vi "UI Main.vi"() -> ()   [LabVIEW 2018]
doc: "Main user interface VI running on HMI"
uses:
  Controls/Control Mode.ctl
  Controls/Parameters.ctl
  Controls/Sensor CalPara.ctl
  Controls/UI Controls.ctl
  Support/Message Queue/Message.ctl
  <vilib>/Utility/miscctls.llb/LVBoundsTypeDef.ctl
  Controls/Pumps Command.ctl
  Support/Message Queue/Message Cluster.ctl
  Controls/Calibration Cluster.ctl
  Controls/ConfigCalibration.ctl
  Controls/All Control Configuration Values.ctl
  Controls/Machine State.ctl
  Controls/TWT State.ctl
  Controls/OT State.ctl
  Controls/IT State.ctl
  Controls/BR State.ctl
  Controls/Pumps State.ctl
  Controls/DL State.ctl
  Controls/Clamp State.ctl
  Controls/Clean State.ctl
  Controls/Status Message.ctl
  Globals/Global - All UI Loop Stop.vi
  Globals/Global - UI Stream and Variable Connections.vi
  Globals/Global - Configuration Options.vi
  support/User Event - Stop/User Event - Stop.lvlib
  support/Message Queue/Message Queue.lvlib
panel:
  out "Temperature 8":u16(ring)
  out "Temperature 7":u16(ring)
  out "Temperature 6":u16(ring)
  in  "AB Valve":dbl(slide) scale=0.0..100.0
  in  "Horizontal Pointer Slide":dbl(slide) caption="Bleed Valve" scale=0.0..100.0
  in  "TC Valve":dbl(slide) scale=0.0..100.0
  out "Temp 11":dbl format="%.1f %"
  out "Pressure 7":dbl format="%.1f PSI"
  out "Temp 12":dbl format="%.1f F"
  out "Temp 10":dbl format="%.1f F"
  out "Pressure 5":dbl format="%.1f PSI"
  out "Temp 9":dbl format="%.1f F"
  out "RPM 2":dbl format="%.1f RPM"
  out "Temp 8":dbl format="%.1f F"
  out "Pressure 4":dbl format="%.1f PSI"
  out "Temp 7":dbl format="%.1f F"
  out "Temp 6":dbl format="%.1f F"
  out "Temp 5":dbl format="%.1f F"
  out "Temp 4":dbl format="%.1f F"
  out "Pressure 3":dbl format="%.1f PSI"
  out "Temp 3":dbl format="%.1f F"
  out "Temp 2":dbl format="%.1f F"
  in  "Checkbox 5":bool
  in  "Bearing Lube Switch 2":bool caption="Bearing Cooling"
  in  "Bearing Lube Switch":bool caption="Bearing Lube"
  out "RPM":dbl format="%.1f RPM"
  out "Pressure":dbl format="%.1f PSI"
  out "Temp":dbl format="%.1f F"
  in  "Checkbox 4":bool
  in  "Triplex Pump Switch":bool caption="Triplex Pump"
  in  "Oil Circ Switch":bool caption="Oil Circ"
  in  "Heater Switch":bool caption="Water Heater"
  out "Temperature 5":u16(ring)
  out "CRIO Version":string="V4.0" caption="CRIO:"
  out "HMI Version":string="V4.0" caption="HMI:"
  out "Temperature 2":u16(ring)
  in  "Tab Control":T1(tab)
  out "Pump 5":u16(ring)
  out "Pump 4":u16(ring)
  out "Pump 3":u16(ring)
  out "Pump 2":u16(ring)
  out "Oil Temperature Sid B (Deg F)":dbl(knob) scale=50.0..300.0 scale format="%#.1f"
  out "HPU Ambient\nTemperature (Deg F)":dbl(slide) scale=0.0..100.0 scale format="%#_1f"
  out "Oil Temperature Sid A (Deg F)":dbl(knob) scale=50.0..300.0 scale format="%#.1f"
  out "Pump 1":u16(ring)
  out "Temperature 3":u16(ring)
  out "Sensor CalPara":T2={"Body CalPara"={"Slope"=62500.0, "Intercept"=-250.0}, "US CalPara"={"Slope"=62500.0, "Intercept"=-250.0}} {"US CalPara"."Intercept" format="%.6f"; "US CalPara"."Slope" format="%.6f"; "Body CalPara"."Intercept" format="%.6f"; "Body CalPara"."Slope" format="%.6f"}
  in  "Stop":bool
  out "Running":bool
  out "Connection":bool
  out "data":T4
  out "Triplex Pump":bool
  out "Power Pack":bool
  out "Any Door":bool
  out "Platform Locks\nEngaged":bool
  out "Platform Locks\nDisengaged":bool
  out "Temperature 4":u16(ring)
  out "Mandrel Temp":dbl format="%.1f"
  out "Brg Mandrel Temp":dbl format="%.1f"
  out "Ambient Temp":dbl format="%.1f"
  out "Vessel Temp":dbl format="%.1f"
  out "Temperature":u16(ring)
  out "SW":dbl
  out "SE":dbl
  out "NW":dbl
  out "NE":dbl
  out "Cylinder Force (lbf)":cluster{i32, "number: 0 to 1":dbl}[](graph)
  in  "US CAL":bool caption="Sensor 1"
  in  "Body CAL":bool caption="Sensor 1"
  out "Free Memory (bytes)":dbl(graph)
  out "CPU Usage (%)":dbl(graph)
  in  "Status ListBox":i32(listbox)
  in  "Triplex Pump":dbl(slide) caption="Set Speed" scale=0.0..100.0
  # "Pressure Sensors"
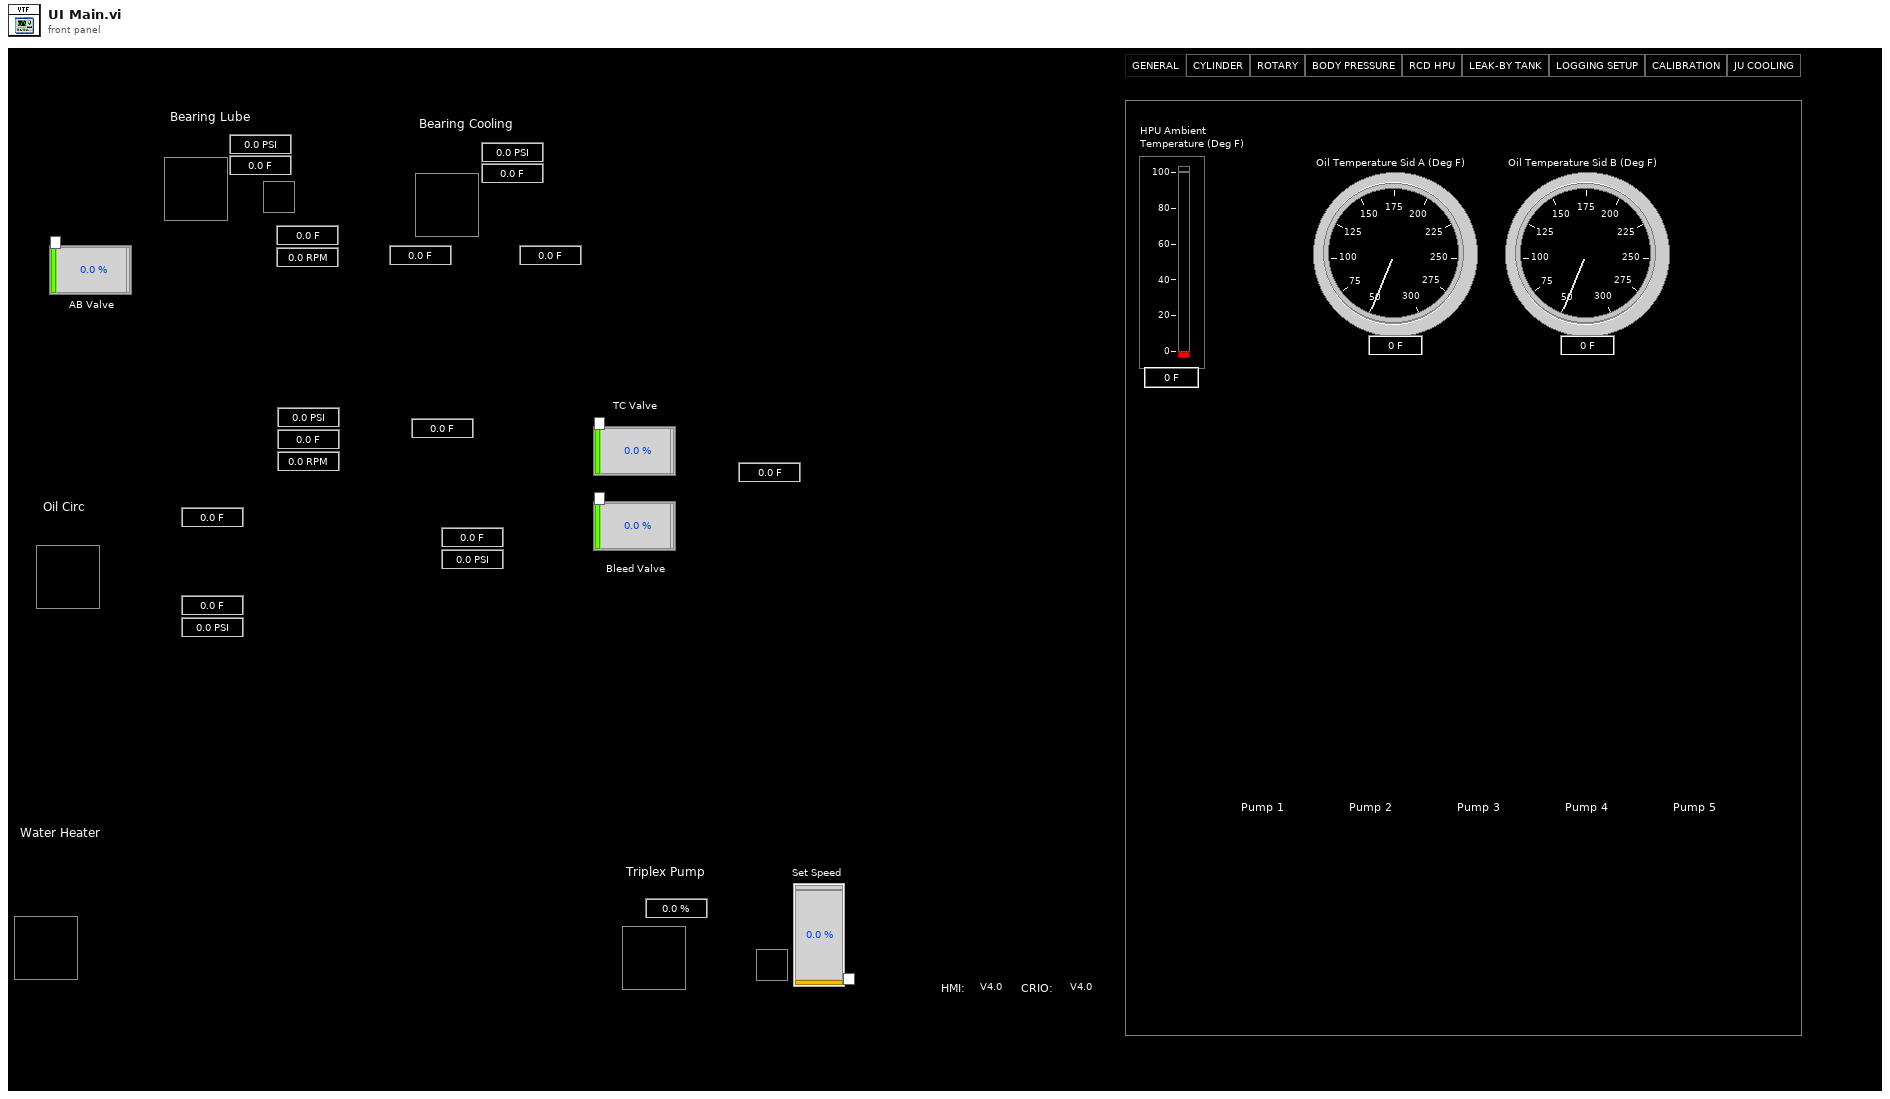
[diagram p1: front panel]
types:
  T1 = enum32{"GENERAL", "CYLINDER", "ROTARY", "BODY PRESSURE", "RCD HPU", "LEAK-BY TANK", "LOGGING SETUP", "CALIBRATION", "JU COOLING"}
  T2 = typedef "Parameters.ctl" = cluster{"Body CalPara":T3, "US CalPara":T3}
  T3 = typedef "Sensor CalPara.ctl" = cluster{"Slope":dbl, "Intercept":dbl}
  T4 = typedef "Control Mode.ctl" = enum16{"Skid Manual", "Computer Manual", "Step Automated", "Fully Automated"}
  T5 = typedef "UI Controls.ctl" = cluster{"Stop":refnum<vi>, "Pump 1":refnum<vi>, "Pump 2":refnum<vi>, "Pump 3":refnum<vi>, "Pump 4":refnum<vi>, "Pump 5":refnum<vi>}
  T6 = typedef "Message Queue.lvlib/All Message Queues.ctl" = cluster{"UI":refnum<queue>}
  T7 = typedef "Message Queue.lvlib/Message.ctl" = enum16{"Initialize", "Initialize UI Refs", "Disable Controls", "Enable UI Controls", "Connect RT", "Get Control Mode from RT", "Send Control Mode to UI", "Update Control Mode", "Get Config from RT", "Send Config to UI", "Update Parameters", "Change Parameters", "Calibrate Config", "Update Calibration", "Change Valve State", "Get Valve Status from RT", "Send Valve Status to UI", "Update Valve Status", "Inital UI Values", "Disconnect RT", "Close Connection", "Disconnect UI", "Run Mode", "Stop ALL", "Change Control Mode", "Skid Manual", "Computer Manual", "Step Automated", "Fully Automated", "Reset", "Pumps Command", "Pump State Changed", "Critical Error", "Log-Only Error", "Non-Critical Error", "RT Error", "Update System Status", "Update DI Status", "Clear System Status", "Update Warning", "Clear Warning", "Upate Timeout", "Update Reset Status", "Waiting", "Verify Password", "Manual Cleaning Process", "Update Manual Cleaning Process", "Cal - Body", "Cal - US", "Cal - Update Parameters", "Exit", "---Copy This Frame---"}
  T8 = typedef "LVBoundsTypeDef.ctl" = cluster{"Width":u32, "Height":u32}
  T9 = enum16{"Pump 1", "Pump 2", "Pump 3", "Pump 4", "Pump 5"}
  T10 = typedef "Pumps Command.ctl" = cluster{"Pump":enum16{"Pump 1", "Pump 2", "Pump 3", "Pump 4", "Pump 5"}, "Run/Stop":bool}
  T11 = enum8{"Enabled", "Disabled", "Disabled and Grayed Out"}
  T12 = typedef "Message Queue.lvlib/Message Cluster.ctl" = cluster{"Message":T7, "Message Data":variant}
  T13 = typedef "Calibration Cluster.ctl" = cluster{"CONFIG CALIBRATION":T14, "Calibration Value":dbl}
  T14 = typedef "ConfigCalibration.ctl" = enum16{"CAL STOP", "TWTT OP (IN)", "TWTT PDP (IN)", "DLT OP (IN)", "DLT PDP 01 (IN)", "DLT PDP 02 (IN)", "BR OP (IN)", "BR TWT ALIGN (IN)", "BR DL ALIGN (IN)"}
  T15 = typedef "All Control Configuration Values.ctl" = cluster{"MACHINE STATE":T16}
  T16 = typedef "Machine State.ctl" = cluster{"TWTT STATE":T17, "OT STATE":T18, "IT STATE":T19, "BR STATE":T20, "DLT STATE":T21, "DL STATE":T22, "CLAMP STATE":T23, "CLEAN STATE":T24}
  T17 = typedef "TWT State.ctl" = enum16{"TWTT STOP", "TWTT DRIVE FWD PDP", "TWTT DRIVE BWD PDP", "TWTT BWD 0.256 IN", "TWTT FWD 0.256 IN", "TWT FWD BEFORE SCREW", "SV-5 TWTT FWD TRUE", "SV-5 TWTT FWD FALSE", "SV-6 TWTT BWD TRUE", "SV-6 TWTT BWD FALSE", "TWTT RESET"}
  T18 = typedef "OT State.ctl" = enum16{"OT STOP", "OT ROTATE CW ENG", "OT ROTATE CCW 2.5 REV", "OT ROTATE CW 2.5 REV", "OT CW TIGHTEN PLUG", "SV-2 OT CW TRUE", "SV-2 OT CW FALSE", "SV-2 OT CCW TRUE", "SV-2 OT CCW FALSE"}
  T19 = typedef "IT State.ctl" = enum16{"IT STOP", "IT ROTATE CCW ENG", "IT ROTATE CCW QF1R", "IT CCW ENG & QF1R", "IT ROTATE CCW 2.5 REV", "IT ROTATE CW 2.5 REV", "IT CW TIGHTEN VALVE", "IT CCW PULSE", "SV-1 IT CW TRUE", "SV-1 IT CW FALSE", "SV-1 IT CCW TRUE", "SV-1 IT CCW FALSE"}
  T20 = typedef "BR State.ctl" = enum16{"BR STOP", "BR DRIVE LEFT PDP", "BR LEFT ALIGN TWT", "BR DRIVE RIGHT PDP", "BR RIGHT TO INIT", "BR RIGHT FOR DL", "SV-4 BR RIGHT TRUE", "SV-4 BR RIGHT FALSE", "SV-4 BR LEFT TRUE", "SV-4 BR LEFT FALSE", "BR RESET"}
  T21 = typedef "Pumps State.ctl" = enum16{"Do Nothing", "Run Pump 1", "Run Pump 2", "Run Pump 3", "Run Pump 4", "Run Pump 5", "Stop Pump 1", "Stop Pump 2", "Stop Pump 3", "Stop Pump 4", "Stop Pump 5"}
  T22 = typedef "DL State.ctl" = enum16{"DL STOP", "DL ROTATE CW", "DL ROTATE CCW", "SV-3 DL CW TRUE", "SV-3 DL CW FALSE", "SV-3 DL CCW TRUE", "SV-3 DL CCW FALSE"}
  T23 = typedef "Clamp State.ctl" = enum16{"CLAMP STOP", "CLAMP CLOSE", "CLAMP OPEN"}
  T24 = typedef "Clean State.ctl" = enum16{"CLEAN STOP", "CLEAN CAMERA", "CLEAN THREADS", "CLEAN THREADS MANUAL", "SV-12 H2O PILOT TRUE", "SV-12 H2O PILOT FALSE", "SV-13 CLEAN AIR TRUE", "SV-13 CLEAN AIR FALSE", "SV-15 CLEAN H2O TRUE", "SV-15 CLEAN H2O FALSE"}
  T25 = typedef "Status Message.ctl" = cluster{"Message":string, "Step #":i32, "Start/End":bool}
  T26 = cluster{"CPU Usage":refnum<k21>, "Contiguous Memory":refnum<k21>, "VTF Sensors":refnum<k21>}
  T27 = typedef "VTF Sensors.ctl" = cluster{"TJM Temp":dbl, "BrgM Temp":dbl, "Ambient Temp":dbl, "Vessel Temp":dbl}
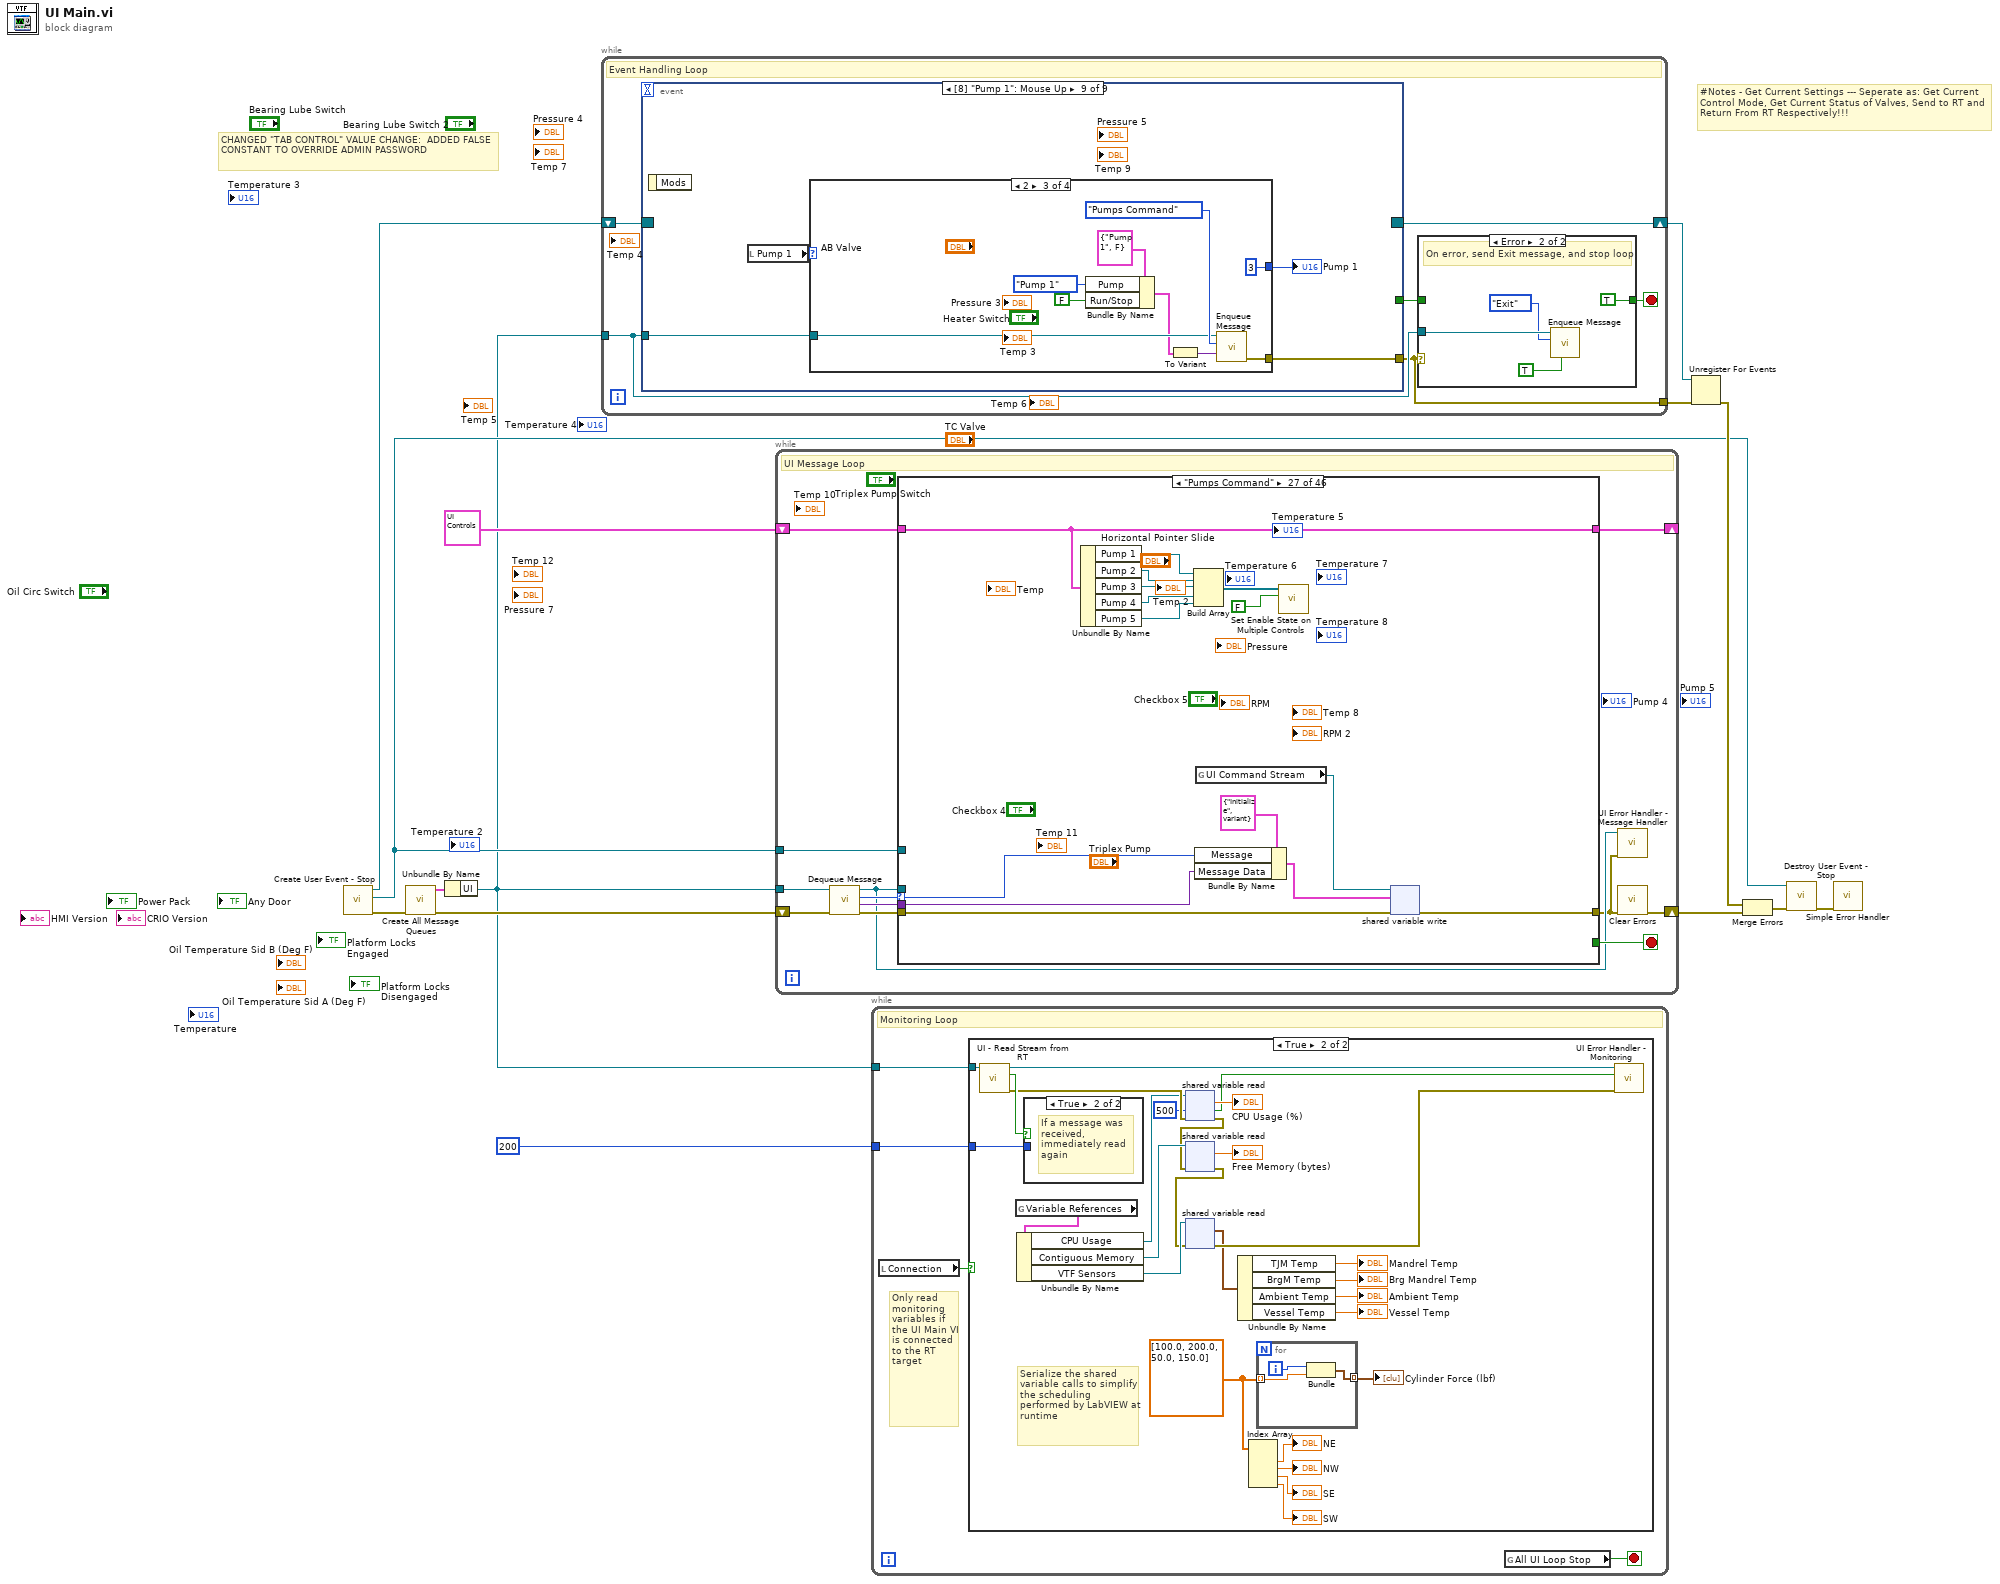
[diagram p0: block diagram]
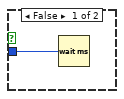
[diagram p3: hidden frame]
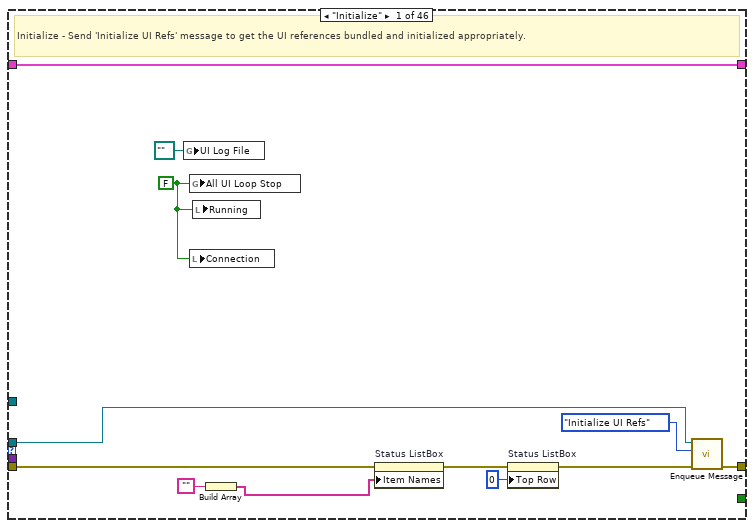
[diagram p4: hidden frame]
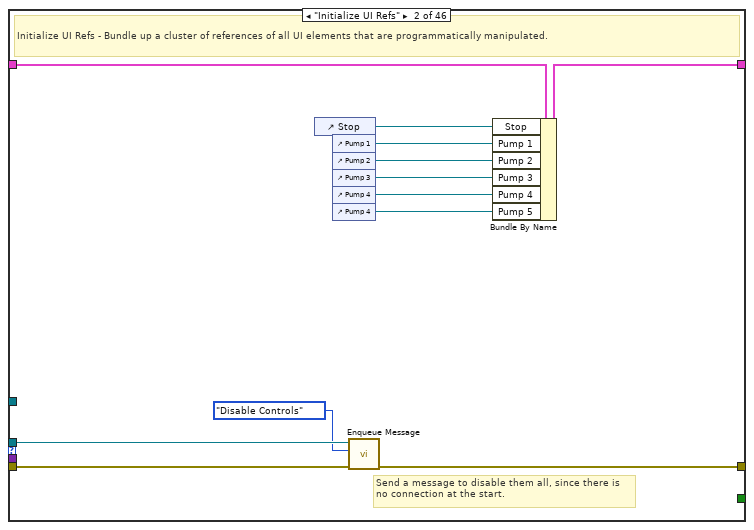
[diagram p5: hidden frame]
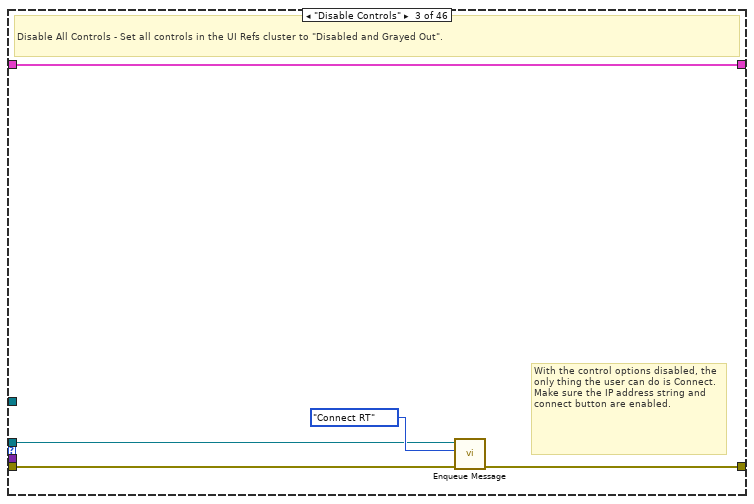
[diagram p6: hidden frame]
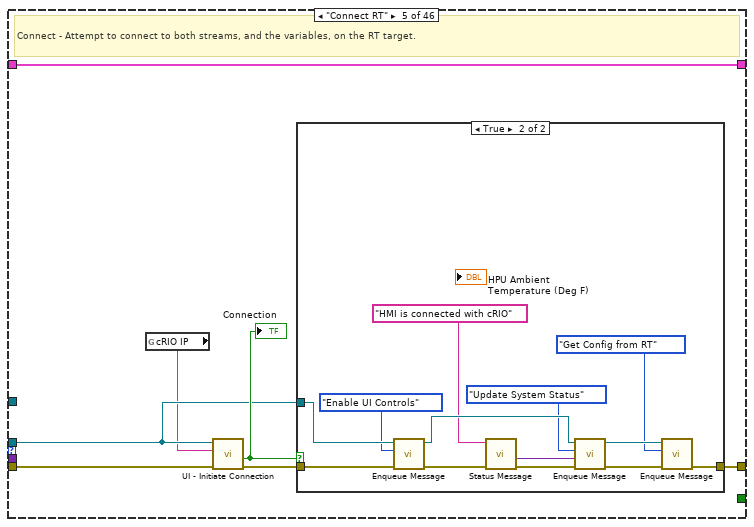
[diagram p8: hidden frame]
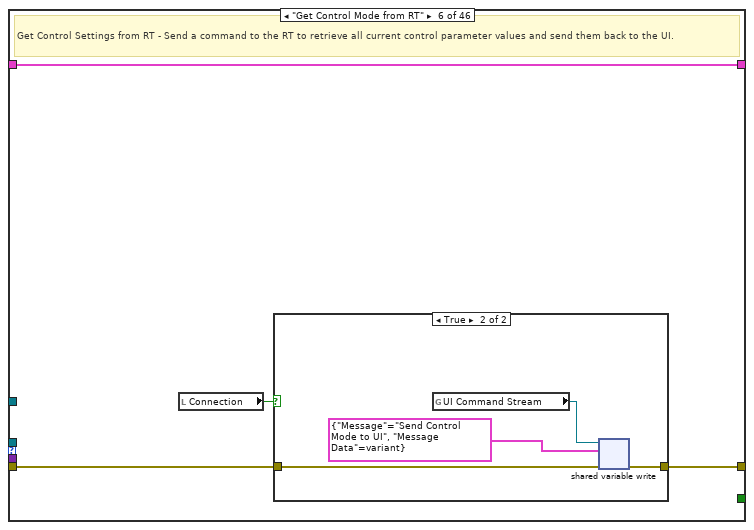
[diagram p10: hidden frame]
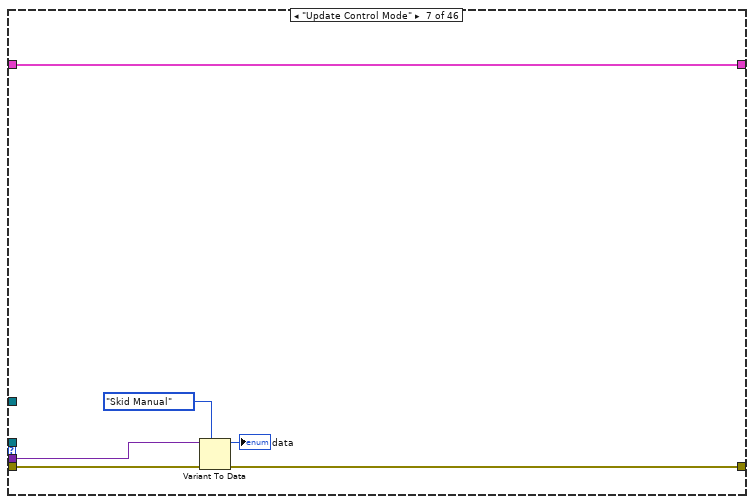
[diagram p12: hidden frame]
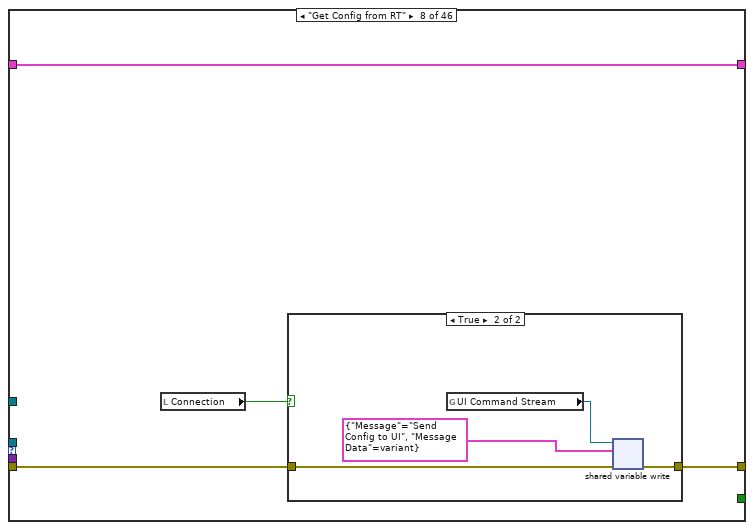
[diagram p13: hidden frame]
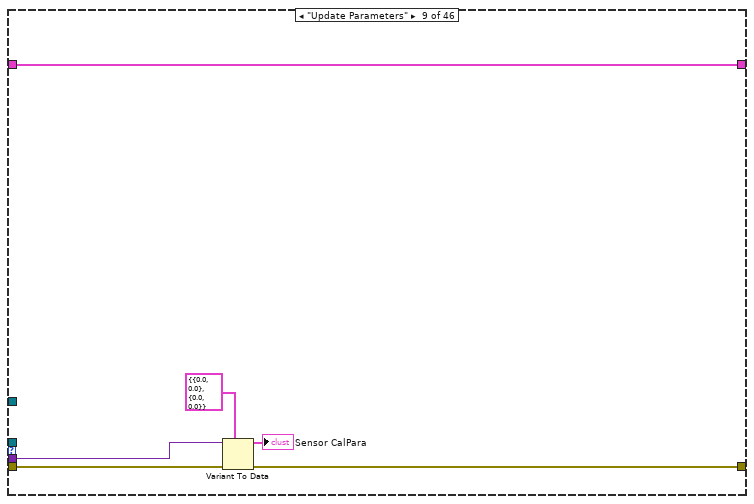
[diagram p15: hidden frame]
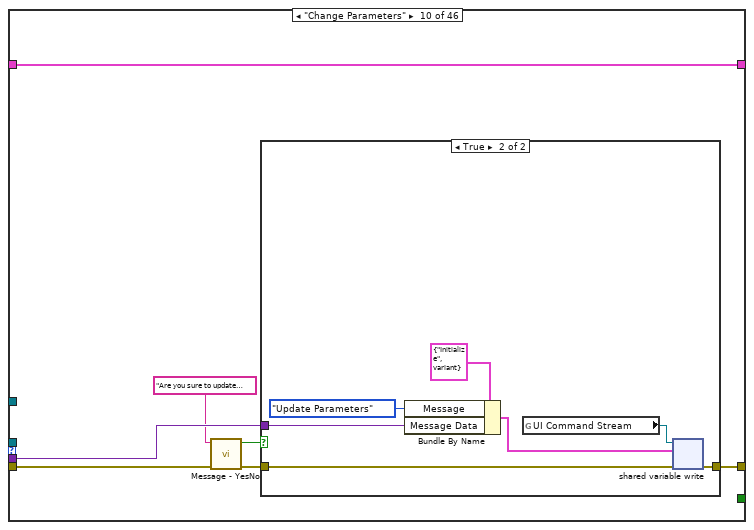
[diagram p16: hidden frame]
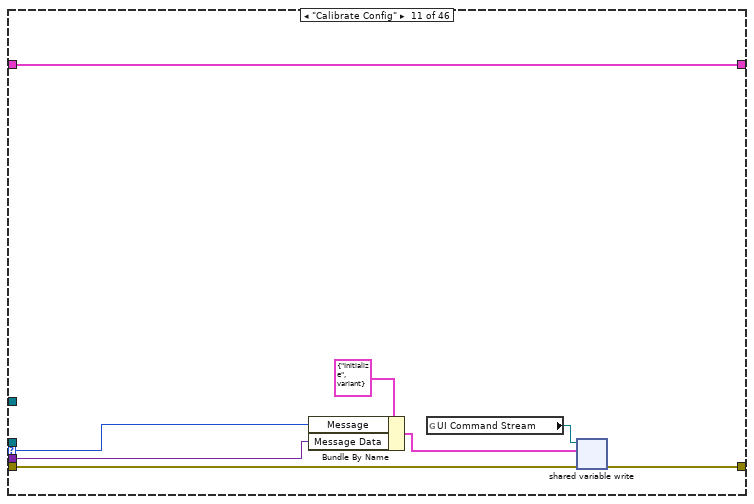
[diagram p18: hidden frame]
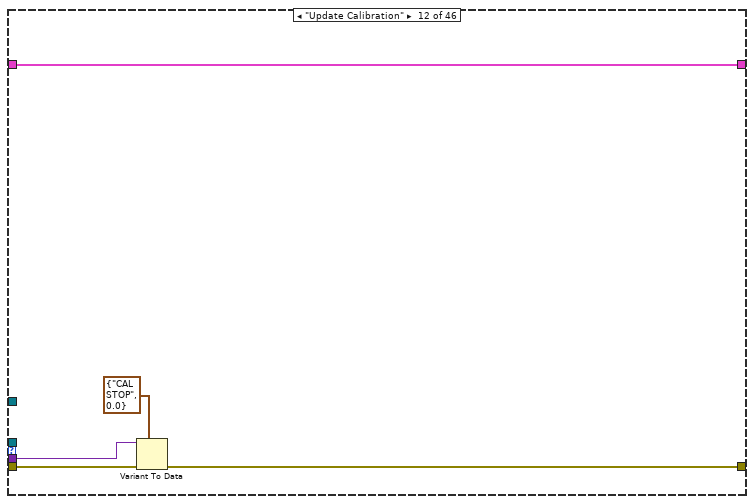
[diagram p19: hidden frame]
diagram:
  # "CHANGED \"TAB CONTROL\" VALUE CHANGE:  ADDED FALSE CONSTANT TO OVERRIDE ADMIN PASSWORD"
  # "#Notes - Get Current Settings --- Seperate as: Get Current Control Mode, Get Current Status of Valves, Send to RT and Return From RT Respectively!!!"
  n1 = call "Create User Event - Stop.vi"() -> ("error out"=w14:errorcluster, "User Event - Stop"=w3:refnum<user-event>, "Stop Event Registration Refnum"=w10:refnum<event-registration>)  [unwired: 9 in]
  n2 = call "Create All Message Queues.vi"("error in (no error)"=w14) -> ("error out"=w12:errorcluster, "Message Queues out"=w13:T6)  [unwired: 9 in]
  n3 = Unbundle By Name(w13) -> ("UI"=w1:refnum<queue>)
  n4 = while {
    tunnel: w1 -> [w20]
    tunnel: [w17] -> w8
    shift-right: [w15] -> w7
    shift-left: w10 -> [w16]
    stop <- w19 stop-if-true
    # "Event Handling Loop"
    n5 = event shown="[8] \"Pump 1\": Mouse Up" {
      selector: w16 -> [_ _ _ _ _ _ _ _ _]
      dyn-events: [_ _ _ _ _ _ _ _ _] -> w15
      timeout: _ -> [_ _ _ _ _ _ _ _ _]
      tunnel: w20 -> [w27 _ w47 _ _ _ w60 w63 w67]
      tunnel: [w26 w32 w46 _ _ _ w59 w62 w66] -> w17
      tunnel: [_ _ _ TRUE _ _ _ _ _] -> w18
      event "Stop": Value Change {
        n6 = event-data() -> ()  [unwired: 1 in, 1 out]
        n7 = call "Enqueue Message.vi"("Message"=Message."Stop ALL", "Message Queue"=w27) -> ("error out"=w26:errorcluster)  [unwired: 8 in, 1 out]
      }
      event "Tab Control": Value Change {
        n8 = event-data() -> ("CtlRef"=w31:refnum<vi>, "NewVal"=w29:T1)  [unwired: 1 in]
        n9 = property class="TabCtl (strict)"(reference=w31) -> (error out=w33:errorcluster, "Pages"=w30:refnum<vi>[])  [unwired: 1 in, 1 out]
        n10 = for {
          tunnel: w33 -> [w38]
          tunnel: [w37] -> w32
          tunnel: w30 -> [w35] mode=indexing
          tunnel: w29 -> [w34]
          i -> [w36]
          n11 = Equal?(x=w34, y=w36) -> (x = y?=w42:bool)
          n12 = Select(t=u32 0, s=w42, f=u32 6579300) -> (s? t:f=w39:u32)
          n13 = property class="Page"(reference=w35, error in=w38, "BG Color"=w39) -> (error out=w37:errorcluster)  [unwired: 1 out]
        }
      }
      event Panel Close? {
        w43 = TRUE  # Priority Message
        n14 = event-data() -> ()  [unwired: 1 in, 1 out]
        n15 = call "Enqueue Message.vi"("Priority Message? (F)"=w43, "Message"=Message."Exit", "Message Queue"=w47) -> ("error out"=w46:errorcluster)  [unwired: 7 in, 1 out]
        n16 = event-data("Discard?"=TRUE) -> ()  [unwired: 1 in, 1 out]
      }
      event User Event {
        # "The Message Handling Loop processed an \"Exit\" message, which fired this event to stop the Event Handling Loop."
        n17 = event-data() -> ()  [unwired: 1 in, 1 out]
      }
      event "Stop": Mouse Enter {
        n18 = event-data() -> ("CtlRef"=w51:refnum<vi>)  [unwired: 1 in]
        n19 = property class="Bool"(reference=w51) -> (reference out=w49:refnum<vi>, "DisabledEnum"=w50:T11)  [unwired: 1 in, 1 out]
        n20 = case shown="\"Enabled\", Default" w50 {
          tunnel: w49 -> [w52 _ _]
          frame "Enabled", Default {
            n21 = property class="Bool"(reference=w52, "Button Size"=T8 {"Width"=136, "Height"=57}) -> ()  [unwired: 1 in, 2 out]
          }
          frame "Disabled" {
          }
          frame "Disabled and Grayed Out" {
          }
        }
      }
      event "Stop": Mouse Leave {
        n22 = event-data() -> ("CtlRef"=w56:refnum<vi>)  [unwired: 1 in]
        n23 = property class="Bool"(reference=w56) -> (reference out=w54:refnum<vi>, "DisabledEnum"=w55:T11)  [unwired: 1 in, 1 out]
        n24 = case shown="\"Enabled\", Default" w55 {
          tunnel: w54 -> [w57 _ _]
          frame "Enabled", Default {
            n25 = property class="Bool"(reference=w57, "Button Size"=T8 {"Width"=135, "Height"=56}) -> ()  [unwired: 1 in, 2 out]
          }
          frame "Disabled" {
          }
          frame "Disabled and Grayed Out" {
          }
        }
      }
      event "Body CAL": Value Change {
        n26 = event-data() -> ()  [unwired: 1 in, 1 out]
        n27 = call "Enqueue Message.vi"("Message"=Message."Cal - Body", "Message Queue"=w60) -> ("error out"=w59:errorcluster)  [unwired: 8 in, 1 out]
      }
      event "US CAL": Value Change {
        n28 = event-data() -> ()  [unwired: 1 in, 1 out]
        n29 = call "Enqueue Message.vi"("Message"=Message."Cal - US", "Message Queue"=w63) -> ("error out"=w62:errorcluster)  [unwired: 8 in, 1 out]
      }
      event "Pump 1": Mouse Up {
        n30 = event-data() -> ()  [unwired: 1 in, 1 out]
        n31 = local read "Pump 1"() -> (w68:u16)
        n32 = case shown="2" w68 {
          selector: w68 -> [_ w78 _ w88]
          tunnel: w67 -> [w76 _ w84 _]
          tunnel: [w75 _ w83 _] -> w66
          tunnel: [u16 1 ("Pump 1") w78 u16 3 ("Pump 1") w88] -> w65
          frame 0, Default {
            n33 = Bundle By Name(cluster=T10 {"Pump"=enum."Pump 1", "Run/Stop"=FALSE} ("Pump CMD"), "Pump"=T9."Pump 1", "Run/Stop"=TRUE) -> (w69:T10)
            n34 = To Variant(anything=w69) -> (Variant=w73:variant)
            n35 = call "Enqueue Message.vi"("Message Data"=w73, "Message"=Message."Pumps Command", "Message Queue"=w76) -> ("error out"=w75:errorcluster)  [unwired: 7 in, 1 out]
          }
          frame 1 {
          }
          frame 2 {
            n36 = Bundle By Name(cluster=T10 {"Pump"=enum."Pump 1", "Run/Stop"=FALSE} ("Pump CMD"), "Pump"=T9."Pump 1", "Run/Stop"=FALSE) -> (w79:T10)
            n37 = To Variant(anything=w79) -> (Variant=w85:variant)
            n38 = call "Enqueue Message.vi"("Message Data"=w85, "Message"=Message."Pumps Command", "Message Queue"=w84) -> ("error out"=w83:errorcluster)  [unwired: 7 in, 1 out]
          }
          frame 3 {
          }
        }
        "Pump 1" <- w65
      }
    }
    n39 = case shown="Error" w17 {
      tunnel: w20 -> [_ w25]
      tunnel: [w21 TRUE] -> w19
      tunnel: w18 -> [w21 _]
      frame No Error {
      }
      frame Error {
        # "On error, send Exit message, and stop loop."
        n40 = call "Enqueue Message.vi"("Priority Message? (F)"=TRUE, "Message"=Message."Exit", "Message Queue"=w25) -> ()  [unwired: 7 in, 2 out]
      }
    }
  }
  n41 = while {
    tunnel: w1 -> [w100]
    shift-right: [w95] -> w9
    shift-left: w12 -> [w99]
    shift-right: [w93] -> _
    shift-left: T5 {"Stop"=refnum, "Pump 1"=refnum, "Pump 2"=refnum, "Pump 3"=refnum, "Pump 4"=refnum, "Pump 5"=refnum} ("UI Controls") -> [w94]
    tunnel: w3 -> [w89]
    stop <- w92 stop-if-true
    # "UI Message Loop"
    n42 = call "Dequeue Message.vi"("error in (no error)"=w99, "Message Queue"=w100) -> ("error out"=w96:errorcluster, "Message Data"=w97:variant, "Message"=w98:T7, "dup Message Queue"=w91:refnum<queue>)  [unwired: 6 in]
    n43 = case shown="\"Pumps Command\"" w98 {
      selector: w98 -> [_ _ _ _ _ _ _ _ _ _ w198 _ _ _ _ _ _ _ _ w256 w269 w274 _ _ _ _ w302 _ _ _ _ _ w342 _ _ _ _ w361 w369 w377 w385 _ _ w428 _ _]
      tunnel: w97 -> [_ _ _ _ _ _ w164 _ w181 w188 w204 w209 _ _ _ w217 _ _ _ _ _ w275 _ w283 w289 w295 w301 _ _ _ _ w339 w343 _ _ _ _ w362 w370 w378 w386 _ _ w429 _ _]
      tunnel: w96 -> [w101 w121 w127 w130 w135 w155 w166 w169 w180 w184 w202 w207 w212 w214 w216 w220 w224 w234 w253 w260 w268 w280 w281 w287 w293 w299 w304 w316 w318 w321 w323 w338 w348 w352 w354 w356 w358 w367 w375 w383 w391 w399 w417 w431 w443 w460]
      tunnel: [w105 w120 w126 w130 w137 w154 w165 w168 w179 w187 w203 w206 w212 w214 w216 w219 w223 w233 w253 w259 w267 w278 w281 w286 w292 w298 w303 w316 w318 w321 w323 w324 w346 w351 w354 w356 w358 w365 w373 w381 w389 w394 w412 w430 w436 w460] -> w90
      tunnel: w94 -> [w111 w124 w125 w131 w132 w156 w167 w171 w182 w189 w205 w210 w211 w213 w215 w221 w228 w229 w252 w263 w266 w279 w282 w288 w294 w300 w315 w317 w319 w320 w322 w340 w347 w353 w355 w357 w359 w366 w374 w382 w390 w400 w418 w435 w446 w461]
      tunnel: [w111 w123 w125 w131 w132 w156 w167 w171 w182 w189 w205 w210 w211 w213 w215 w221 w228 w229 w252 w263 w266 w279 w282 w288 w294 w300 w315 w317 w319 w320 w322 w340 w347 w353 w355 w357 w359 w366 w374 w382 w390 w400 w418 w435 w446 w461] -> w93
      tunnel: w91 -> [w104 w122 w128 _ w134 _ _ _ _ _ _ _ _ _ _ _ w222 w230 _ _ _ _ _ w285 w291 w297 _ _ _ _ _ _ _ _ _ _ _ _ _ _ _ w392 w410 _ w444 _]
      tunnel: [_ _ _ _ _ _ _ _ _ _ _ _ _ _ _ _ _ _ _ _ _ _ _ _ _ _ _ _ _ _ _ _ _ _ _ _ _ _ _ _ _ _ _ _ TRUE _] -> w92
      tunnel: w89 -> [_ _ _ _ _ _ _ _ _ _ _ _ _ _ _ _ _ _ _ _ _ _ _ _ _ _ _ _ _ _ _ _ _ _ _ _ _ _ _ _ _ _ _ _ w441 _]
      frame "Initialize" {
        w110 = FALSE ("All UI Loop Stop")
        # "Initialize - Send 'Initialize UI Refs' message to get the UI references bundled and initialized appropriately."
        n44 = global write "Global - Configuration Options.vi" "UI Log File"(path "" ("UI Log File")) -> ()
        n45 = global write "Global - All UI Loop Stop.vi" "All UI Loop Stop"(w110) -> ()
        n46 = local write "Connection"(w110) -> ()
        n47 = local write "Running"(w110) -> ()
        n48 = Build Array("") -> (w102:string[])
        n49 = property on="Status ListBox" class="LstBox (strict)"(error in=w101, "Item Names"=w102) -> (error out=w103:errorcluster)  [unwired: 1 in, 1 out]
        n50 = property on="Status ListBox" class="LstBox (strict)"(error in=w103, "Top Row"=0) -> (error out=w106:errorcluster)  [unwired: 1 in, 1 out]
        n51 = call "Enqueue Message.vi"("error in (no error)"=w106, "Message"=Message."Initialize UI Refs", "Message Queue"=w104) -> ("error out"=w105:errorcluster)  [unwired: 7 in, 1 out]
      }
      frame "Initialize UI Refs" {
        # "Send a message to disable them all, since there is no connection at the start."
        # "Initialize UI Refs - Bundle up a cluster of references of all UI elements that are programmatically manipulated."
        n52 = control-ref of="Stop"() -> (w118:refnum<vi>)
        n53 = control-ref of="Pump 1"() -> (w117:refnum<vi>)
        n54 = control-ref of="Pump 2"() -> (w116:refnum<vi>)
        n55 = control-ref of="Pump 3"() -> (w115:refnum<vi>)
        n56 = control-ref of="Pump 4"() -> (w114:refnum<vi>)
        n57 = control-ref of="Pump 4"() -> (w113:refnum<vi>)
        n58 = call "Enqueue Message.vi"("error in (no error)"=w121, "Message"=Message."Disable Controls", "Message Queue"=w122) -> ("error out"=w120:errorcluster)  [unwired: 7 in, 1 out]
        n59 = Bundle By Name(cluster=w124, "Stop"=w118, "Pump 1"=w117, "Pump 2"=w116, "Pump 3"=w115, "Pump 4"=w114, "Pump 5"=w113) -> (w123:T5)
      }
      frame "Disable Controls" {
        # "With the control options disabled, the only thing the user can do is Connect. Make sure the IP address string and connect button are enabled."
        # "Disable All Controls - Set all controls in the UI Refs cluster to \"Disabled and Grayed Out\"."
        n60 = call "Enqueue Message.vi"("error in (no error)"=w127, "Message"=Message."Connect RT", "Message Queue"=w128) -> ("error out"=w126:errorcluster)  [unwired: 7 in, 1 out]
      }
      frame "Enable UI Controls" {
        # "Once connected, the user shouldn't be able to change the connection settings unless he gets disconnected."
        # "Enable Configuration Controls - After successful connection, ensure appropriate controls are enabled."
      }
      frame "Connect RT" {
        # "Connect - Attempt to connect to both streams, and the variables, on the RT target."
        n61 = global read "Global - Configuration Options.vi" "cRIO IP"() -> (w133:string)
        n62 = call "UI - Initiate Connection.vi"("error in"=w135, "Controller Address"=w133, "Message Queue"=w134) -> ("error out"=w138:errorcluster, "Connected?"=w136:bool)  [unwired: 7 in]
        "Connection" <- w136
        n63 = case shown="True" w136 {
          tunnel: w138 -> [w139 w150]
          tunnel: [w139 w141] -> w137
          tunnel: w134 -> [_ w152]
          frame False {
          }
          frame True {
            n64 = call "Enqueue Message.vi"("error in (no error)"=w150, "Message"=Message."Enable UI Controls", "Message Queue"=w152) -> ("error out"=w144:errorcluster, "dup Message Queue"=w149:refnum<queue>)  [unwired: 7 in]
            n65 = call "Status Message.vi"("Error In"=w144, "Message"="HMI is connected with cRIO") -> ("Error Out"=w147:errorcluster, "Status"=w145:variant)  [unwired: 7 in]
            n66 = call "Enqueue Message.vi"("error in (no error)"=w147, "Message Data"=w145, "Message"=Message."Update System Status", "Message Queue"=w149) -> ("error out"=w142:errorcluster, "dup Message Queue"=w143:refnum<queue>)  [unwired: 6 in]
            n67 = call "Enqueue Message.vi"("error in (no error)"=w142, "Message"=Message."Get Config from RT", "Message Queue"=w143) -> ("error out"=w141:errorcluster)  [unwired: 7 in, 1 out]
          }
        }
      }
      frame "Get Control Mode from RT" {
        # "Get Control Settings from RT - Send a command to the RT to retrieve all current control parameter values and send them back to the UI."
        n68 = local read "Connection"() -> (w153:bool)
        n69 = case shown="True" w153 {
          tunnel: w155 -> [w157 w161]
          tunnel: [w157 w160] -> w154
          frame False {
            # "Don't bother trying to send a message to the RT system if UI Main VI isn't even connected"
          }
          frame True {
            n70 = global read "Global - UI Stream and Variable Connections.vi" "UI Command Stream"() -> (w158:refnum<k21>)
            n71 = shared-variable-write(w158, w161, T12 {"Message"=enum."Send Control Mode to UI", "Message Data"=variant} ("data in")) -> (w160:errorcluster)  [unwired: 1 in, 2 out]
          }
        }
      }
      frame "Update Control Mode" {
        n72 = Variant To Data(error in=w166, type=Control_Mode."Skid Manual" ("Control Mode"), Variant=w164) -> (data=→"data":T4, error out=w165:errorcluster)
      }
      frame "Get Config from RT" {
        n73 = local read "Connection"() -> (w170:bool)
        n74 = case shown="True" w170 {
          tunnel: w169 -> [w172 w176]
          tunnel: [w172 w175] -> w168
          frame False {
            # "Don't bother trying to send a message to the RT system if UI Main VI isn't even connected"
          }
          frame True {
            n75 = global read "Global - UI Stream and Variable Connections.vi" "UI Command Stream"() -> (w173:refnum<k21>)
            n76 = shared-variable-write(w173, w176, T12 {"Message"=enum."Send Config to UI", "Message Data"=variant} ("data in")) -> (w175:errorcluster)  [unwired: 1 in, 2 out]
          }
        }
      }
      frame "Update Parameters" {
        n77 = Variant To Data(error in=w180, type=T2 {"Body CalPara"={"Slope"=0.0, "Intercept"=0.0}, "US CalPara"={"Slope"=0.0, "Intercept"=0.0}} ("PARAMETERS"), Variant=w181) -> (data=→"Sensor CalPara":T2, error out=w179:errorcluster)
      }
      frame "Change Parameters" {
        n78 = call "Message - YesNo.vi"("error in"=w184, "Message In"="Are you sure to update configurations?") -> ("error out"=w183:errorcluster, "Good?"=w185:bool)  [unwired: 8 in]
        n79 = case shown="True" w185 {
          tunnel: w188 -> [_ w193]
          tunnel: [w190 w192] -> w187
          tunnel: w183 -> [w190 w191]
          frame False {
          }
          frame True {
            n80 = Bundle By Name(cluster=T12 {"Message"=enum."Initialize", "Message Data"=variant} ("input cluster"), "Message"=Message."Update Parameters", "Message Data"=w193) -> (w195:T12)
            n81 = global read "Global - UI Stream and Variable Connections.vi" "UI Command Stream"() -> (w197:refnum<k21>)
            n82 = shared-variable-write(w197, w191, w195) -> (w192:errorcluster)  [unwired: 1 in, 2 out]
          }
        }
      }
      frame "Calibrate Config" {
        n83 = Bundle By Name(cluster=T12 {"Message"=enum."Initialize", "Message Data"=variant} ("input cluster"), "Message"=w198, "Message Data"=w204) -> (w199:T12)
        n84 = global read "Global - UI Stream and Variable Connections.vi" "UI Command Stream"() -> (w201:refnum<k21>)
        n85 = shared-variable-write(w201, w202, w199) -> (w203:errorcluster)  [unwired: 1 in, 2 out]
      }
      frame "Update Calibration" {
        n86 = Variant To Data(error in=w207, type=T13 {"CONFIG CALIBRATION"=enum."CAL STOP", "Calibration Value"=0.0} ("Calibration Cluster"), Variant=w209) -> (error out=w206:errorcluster)  [unwired: 1 out]
      }
      frame "Get Valve Status from RT" {
      }
      frame "Send Valve Status to UI" {
      }
      frame "Update Valve Status" {
      }
      frame "Inital UI Values" {
        n87 = Variant To Data(error in=w220, type=T15 {"MACHINE STATE"={"TWTT STATE"=enum."TWTT STOP", "OT STATE"=enum."OT STOP", "IT STATE"=enum."IT STOP", "BR STATE"=enum."BR STOP", "DLT STATE"=enum."Do Nothing", "DL STATE"=enum."DL STOP", "CLAMP STATE"=enum."CLAMP STOP", "CLEAN STATE"=enum."CLEAN STOP"}} ("All Control Configuration Values"), Variant=w217) -> (error out=w219:errorcluster)  [unwired: 1 out]
      }
      frame "Disconnect RT" {
        n88 = call "Enqueue Message.vi"("error in (no error)"=w224, "Message"=Message."Disable Controls", "Message Queue"=w222) -> ("error out"=w223:errorcluster)  [unwired: 7 in, 1 out]
        n89 = global read "Global - UI Stream and Variable Connections.vi" "UI Command Stream"() -> (w227:refnum<k21>)
        n90 = global read "Global - UI Stream and Variable Connections.vi" "RT Message Stream"() -> (w226:refnum<k21>)
        n91 = Destroy Stream Endpoint(11:w226) -> ()  [unwired: 1 in, 1 out]
        n92 = Destroy Stream Endpoint(11:w227) -> ()  [unwired: 1 in, 1 out]
      }
      frame "Close Connection" {
        n93 = flat-sequence {
          tunnel: w234 -> [w240]
          tunnel: [w240] -> w232
          tunnel: [w238] -> w231
          tunnel: w230 -> [w238]
          tunnel: [w242] -> w233
          tunnel: w232 -> [w245]
          tunnel: w231 -> [w241]
          frame #0 {
            n94 = global read "Global - UI Stream and Variable Connections.vi" "UI Command Stream"() -> (w236:refnum<k21>)
            n95 = global read "Global - UI Stream and Variable Connections.vi" "RT Message Stream"() -> (w237:refnum<k21>)
            n96 = global read "Global - UI Stream and Variable Connections.vi" "Variable References"() -> (w235:T26)
            n97 = local write "Connection"(FALSE ("Connected?")) -> ()
            n98 = Destroy Stream Endpoint(11:w236) -> ()  [unwired: 1 in, 1 out]
            n99 = Destroy Stream Endpoint(11:w237) -> ()  [unwired: 1 in, 1 out]
            n100 = call "Close Variable Connections.vi"("Variable References"=w235) -> ()  [unwired: 11 in]
          }
          frame #1 {
            n101 = call "Message - YesNo.vi"("error in"=w245, "Message In"="Lost connection with cRIO! Try to reconnect?") -> ("error out"=w243:errorcluster, "Good?"=w244:bool)  [unwired: 8 in]
            n102 = case shown="True" w244 {
              tunnel: w243 -> [w247 w250]
              tunnel: [w247 w249] -> w242
              tunnel: w241 -> [_ w248]
              frame False {
              }
              frame True {
                n103 = call "Enqueue Message.vi"("error in (no error)"=w250, "Message"=Message."Initialize", "Message Queue"=w248) -> ("error out"=w249:errorcluster)  [unwired: 7 in, 1 out]
              }
            }
          }
        }
      }
      frame "Disconnect UI" {
      }
      frame "Run Mode" {
        # "Running\nTRUE"
        n104 = To Variant(anything=TRUE ("Fully Automated")) -> (Variant=w255:variant)
        n105 = global read "Global - UI Stream and Variable Connections.vi" "UI Command Stream"() -> (w261:refnum<k21>)
        n106 = Bundle By Name(cluster=T12 {"Message"=enum."Initialize", "Message Data"=variant} ("input cluster"), "Message"=w256, "Message Data"=w255) -> (w257:T12)
        n107 = shared-variable-write(w261, w260, w257) -> (w259:errorcluster)  [unwired: 1 in, 2 out]
        n108 = local write "Running"(TRUE ("Running?")) -> ()
      }
      frame "Stop ALL" {
        n109 = Bundle By Name(cluster=T12 {"Message"=enum."Initialize", "Message Data"=variant} ("input cluster"), "Message"=w269) -> (w270:T12)
        n110 = global read "Global - UI Stream and Variable Connections.vi" "UI Command Stream"() -> (w272:refnum<k21>)
        n111 = global write "Global - Configuration Options.vi" "UI Log File"(path "" ("UI Log File")) -> ()
        n112 = shared-variable-write(w272, w268, w270) -> (w267:errorcluster)  [unwired: 1 in, 2 out]
        "Running" <- FALSE ("Running?")
      }
      frame "Change Control Mode" {
        n113 = Bundle By Name(cluster=T12 {"Message"=enum."Initialize", "Message Data"=variant} ("input cluster"), "Message"=w274, "Message Data"=w275) -> (w273:T12)
        n114 = global read "Global - UI Stream and Variable Connections.vi" "UI Command Stream"() -> (w277:refnum<k21>)
        n115 = shared-variable-write(w277, w280, w273) -> (w278:errorcluster)  [unwired: 1 in, 2 out]
      }
      frame "Skid Manual" {
      }
      frame "Computer Manual" {
        n116 = call "Enqueue Message.vi"("error in (no error)"=w287, "Message Data"=w283, "Message"=Message."Update Control Mode", "Message Queue"=w285) -> ("error out"=w286:errorcluster)  [unwired: 6 in, 1 out]
      }
      frame "Step Automated" {
        n117 = call "Enqueue Message.vi"("error in (no error)"=w293, "Message Data"=w289, "Message"=Message."Update Control Mode", "Message Queue"=w291) -> ("error out"=w292:errorcluster)  [unwired: 6 in, 1 out]
      }
      frame "Fully Automated" {
        n118 = call "Enqueue Message.vi"("error in (no error)"=w299, "Message Data"=w295, "Message"=Message."Update Control Mode", "Message Queue"=w297) -> ("error out"=w298:errorcluster)  [unwired: 6 in, 1 out]
      }
      frame "Pumps Command" {
        n119 = Unbundle By Name(w315) -> ("Pump 1"=w314:refnum<vi>, "Pump 2"=w313:refnum<vi>, "Pump 3"=w312:refnum<vi>, "Pump 4"=w311:refnum<vi>, "Pump 5"=w310:refnum<vi>)
        n120 = Build Array(w314, w313, w312, w311, w310) -> (w309:refnum<vi>[])
        n121 = Bundle By Name(cluster=T12 {"Message"=enum."Initialize", "Message Data"=variant} ("input cluster"), "Message"=w302, "Message Data"=w301) -> (w305:T12)
        n122 = global read "Global - UI Stream and Variable Connections.vi" "UI Command Stream"() -> (w307:refnum<k21>)
        n123 = call "Set Enable State on Multiple Controls.vi"("Enable?"=FALSE, "Controls"=w309) -> ()  [unwired: 10 in]
        n124 = shared-variable-write(w307, w304, w305) -> (w303:errorcluster)  [unwired: 1 in, 2 out]
      }
      frame "Critical Error" {
      }
      frame "Log-Only Error" {
      }
      frame "Non-Critical Error" {
      }
      frame "RT Error" {
      }
      frame "Update System Status" {
        n125 = Variant To Data(error in=w338, type=T25 {"Message"="", "Step #"=0, "Start/End"=FALSE} ("Status Message"), Variant=w339) -> (data=w330:T25, error out=w324:errorcluster)
        n126 = Unbundle By Name(w330) -> ("Message"=w329:string)  [unwired: 2 out]
        n127 = Get Date/Time In Seconds() -> (seconds since 1Jan1904=w334:timestamp)
        n128 = Format Date/Time String(seconds (now)=w334) -> (date/time string=w333:string)  [unwired: 2 in]
        n129 = property on="Status ListBox" class="LstBox (strict)"() -> (error out=w326:errorcluster, "Item Names"=w337:string[])  [unwired: 2 in, 1 out]
        n130 = Concatenate Strings(w333, " - " ("string"), w329) -> (w328:string)
        n131 = Insert Into Array(array=w337, index=0, new element=w328) -> (w336:string[])
        n132 = property on="Status ListBox" class="LstBox (strict)"(error in=w326, "Item Names"=w336) -> (error out=w327:errorcluster)  [unwired: 1 in, 1 out]
        n133 = property on="Status ListBox" class="LstBox (strict)"(error in=w327, "Top Row"=0 ("Active Row:Active Row Number")) -> ()  [unwired: 1 in, 2 out]
      }
      frame "Update DI Status" {
        n134 = Bundle By Name(cluster=T12 {"Message"=enum."Initialize", "Message Data"=variant} ("input cluster"), "Message"=w342, "Message Data"=w343) -> (w341:T12)
        n135 = global read "Global - UI Stream and Variable Connections.vi" "UI Command Stream"() -> (w345:refnum<k21>)
        n136 = shared-variable-write(w345, w348, w341) -> (w346:errorcluster)  [unwired: 1 in, 2 out]
      }
      frame "Clear System Status" {
        n137 = Build Array("") -> (w349:string[])
        n138 = property on="Status ListBox" class="LstBox (strict)"(error in=w352, "Item Names"=w349) -> (error out=w351:errorcluster)  [unwired: 1 in, 1 out]
      }
      frame "Update Warning" {
      }
      frame "Upate Timeout" {
      }
      frame "Update Reset Status" {
      }
      frame "Waiting" {
        n139 = Bundle By Name(cluster=T12 {"Message"=enum."Initialize", "Message Data"=variant} ("input cluster"), "Message"=w361, "Message Data"=w362) -> (w360:T12)
        n140 = global read "Global - UI Stream and Variable Connections.vi" "UI Command Stream"() -> (w364:refnum<k21>)
        n141 = shared-variable-write(w364, w367, w360) -> (w365:errorcluster)  [unwired: 1 in, 2 out]
      }
      frame "Verify Password" {
        n142 = Bundle By Name(cluster=T12 {"Message"=enum."Initialize", "Message Data"=variant} ("input cluster"), "Message"=w369, "Message Data"=w370) -> (w368:T12)
        n143 = global read "Global - UI Stream and Variable Connections.vi" "UI Command Stream"() -> (w372:refnum<k21>)
        n144 = shared-variable-write(w372, w375, w368) -> (w373:errorcluster)  [unwired: 1 in, 2 out]
      }
      frame "Manual Cleaning Process" {
        n145 = Bundle By Name(cluster=T12 {"Message"=enum."Initialize", "Message Data"=variant} ("input cluster"), "Message"=w377, "Message Data"=w378) -> (w376:T12)
        n146 = global read "Global - UI Stream and Variable Connections.vi" "UI Command Stream"() -> (w380:refnum<k21>)
        n147 = shared-variable-write(w380, w383, w376) -> (w381:errorcluster)  [unwired: 1 in, 2 out]
      }
      frame "Update Manual Cleaning Process" {
        n148 = Bundle By Name(cluster=T12 {"Message"=enum."Initialize", "Message Data"=variant} ("input cluster"), "Message"=w385, "Message Data"=w386) -> (w384:T12)
        n149 = global read "Global - UI Stream and Variable Connections.vi" "UI Command Stream"() -> (w388:refnum<k21>)
        n150 = shared-variable-write(w388, w391, w384) -> (w389:errorcluster)  [unwired: 1 in, 2 out]
      }
      frame "Cal - Body" {
        n151 = local read "Sensor CalPara"() -> (w393:T2)
        n152 = Unbundle By Name(w393) -> ("Body CalPara"=w396:T3)
        n153 = call "Sensor Calibration.vi"("error in"=w399, "Old Cal Parameters In"=w396) -> ("error out"=w395:errorcluster, "New Cal Parameters"=w397:T3, "Update"=w398:bool)  [unwired: 7 in]
        n154 = case shown="True" w398 {
          tunnel: w397 -> [_ w406]
          tunnel: w395 -> [w401 w408]
          tunnel: [w401 w407] -> w394
          tunnel: w393 -> [_ w403]
          tunnel: w392 -> [_ w404]
          frame False {
          }
          frame True {
            n155 = Bundle By Name(cluster=w403, "Body CalPara"=w406) -> (w402:T2)
            n156 = local write "Sensor CalPara"(w402) -> ()
            n157 = To Variant(anything=w402) -> (Variant=w405:variant)
            n158 = call "Enqueue Message.vi"("error in (no error)"=w408, "Message Data"=w405, "Message"=Message."Cal - Update Parameters", "Message Queue"=w404) -> ("error out"=w407:errorcluster)  [unwired: 6 in, 1 out]
          }
        }
      }
      frame "Cal - US" {
        n159 = local read "Sensor CalPara"() -> (w411:T2)
        n160 = Unbundle By Name(w411) -> ("US CalPara"=w414:T3)
        n161 = call "Sensor Calibration.vi"("error in"=w417, "Old Cal Parameters In"=w414) -> ("error out"=w413:errorcluster, "New Cal Parameters"=w415:T3, "Update"=w416:bool)  [unwired: 7 in]
        n162 = case shown="True" w416 {
          tunnel: w415 -> [_ w424]
          tunnel: w413 -> [w419 w426]
          tunnel: [w419 w425] -> w412
          tunnel: w411 -> [_ w421]
          tunnel: w410 -> [_ w422]
          frame False {
          }
          frame True {
            n163 = Bundle By Name(cluster=w421, "US CalPara"=w424) -> (w420:T2)
            n164 = local write "Sensor CalPara"(w420) -> ()
            n165 = To Variant(anything=w420) -> (Variant=w423:variant)
            n166 = call "Enqueue Message.vi"("error in (no error)"=w426, "Message Data"=w423, "Message"=Message."Cal - Update Parameters", "Message Queue"=w422) -> ("error out"=w425:errorcluster)  [unwired: 6 in, 1 out]
          }
        }
      }
      frame "Cal - Update Parameters" {
        n167 = Bundle By Name(cluster=T12 {"Message"=enum."Initialize", "Message Data"=variant} ("input cluster"), "Message"=w428, "Message Data"=w429) -> (w432:T12)
        n168 = global read "Global - UI Stream and Variable Connections.vi" "UI Command Stream"() -> (w434:refnum<k21>)
        n169 = shared-variable-write(w434, w431, w432) -> (w430:errorcluster)  [unwired: 1 in, 2 out]
      }
      frame "Exit" {
        # "Stop Event Handling Loop"
        # "Stop UI Message Loop"
        # "Release the UI Message queue reference"
        # "Stop Monitoring Loop"
        # "Exit - Fire the User Event to stop the Event Handling Loop, and toggle the global variable to stop the Monitoring Loop.  This message alone causes all three loops to stop."
        n170 = call "Fire User Event - Stop.vi"("User Event - Stop"=w441) -> ("error out"=w439:errorcluster)  [unwired: 10 in]
        n171 = global write "Global - All UI Loop Stop.vi" "All UI Loop Stop"(TRUE ("Stop Monitoring Loop")) -> ()
        n172 = Release Queue(queue=w444, error in (no error)=w443) -> (error out=w440:errorcluster)  [unwired: 1 in, 2 out]
        n173 = Merge Errors(w439, w440) -> (w438:errorcluster)
        n174 = flat-sequence {
          tunnel: w438 -> [w457]
          tunnel: [w457] -> w437
          frame #0 {
            n175 = global read "Global - UI Stream and Variable Connections.vi" "UI Command Stream"() -> (w459:refnum<k21>)
            n176 = global read "Global - UI Stream and Variable Connections.vi" "RT Message Stream"() -> (w458:refnum<k21>)
            n177 = global read "Global - UI Stream and Variable Connections.vi" "Variable References"() -> (w456:T26)
            n178 = Destroy Stream Endpoint(11:w458) -> ()  [unwired: 1 in, 1 out]
            n179 = call "Close Variable Connections.vi"("Variable References"=w456) -> ()  [unwired: 11 in]
            n180 = Destroy Stream Endpoint(11:w459) -> ()  [unwired: 1 in, 1 out]
          }
        }
        n181 = disable-structure shown="Default" {
          disable-tunnel: w437 -> [w448 w451]
          disable-tunnel: [w447 w449] -> w436
          frame condition #0 (active) {
            n182 = invoke class="VI" method="FP.Close"(error in=w448) -> (error out=w447:errorcluster)  [unwired: 2 in, 2 out]
          }
          frame condition #1 {
            n183 = flat-sequence {
              tunnel: w451 -> [w452]
              tunnel: [w453] -> w450
              tunnel: [w455] -> w449
              tunnel: w450 -> [w455]
              frame #0 {
                n184 = invoke class="VI" method="FP.Close"(error in=w452) -> (error out=w453:errorcluster)  [unwired: 2 in, 2 out]
              }
              frame #1 {
                n185 = Stop(stop? (T)=TRUE) -> ()
              }
            }
          }
        }
      }
      frame Default {
        # "'Default' case only runs if there is a message that isn't defined in any of the other cases.  Output a programming error."
      }
    }
    n186 = call "UI Error Handler - Message Handler.vi"("error in (no error)"=w90, "Message Queue"=w91) -> ()  [unwired: 9 in, 1 out]
    n187 = call <vilib>:"Clear Errors.vi"("error in (no error)"=w90) -> ("error out"=w95:errorcluster)  [unwired: 5 in, 1 out]
  }
  n188 = while {
    tunnel: w1 -> [w465]
    tunnel: u32 200 ("milliseconds to wait") -> [w464]
    stop <- w463 stop-if-true
    # "Only read monitoring variables if the UI Main VI is connected to the RT target"
    # "Monitoring Loop"
    n189 = local read "Connection"() -> (w462:bool)
    n190 = case shown="True" w462 {
      tunnel: w465 -> [_ w492]
      tunnel: w464 -> [_ w490]
      frame False {
      }
      frame True {
        w470 = dbl[] [100.0, 200.0, 50.0, 150.0]
        # "Serialize the shared variable calls to simplify the scheduling performed by LabVIEW at runtime"
        n191 = call "UI - Read Stream from RT.vi"("Message Queue"=w492) -> ("error out"=w489:errorcluster, "Message Received?"=w491:bool, "dup Message Queue"=w481:refnum<queue>)  [unwired: 8 in]
        n192 = global read "Global - UI Stream and Variable Connections.vi" "Variable References"() -> (w483:T26)
        n193 = Unbundle By Name(w483) -> ("CPU Usage"=w488:refnum<k21>, "Contiguous Memory"=w487:refnum<k21>, "VTF Sensors"=w479:refnum<k21>)
        n194 = case shown="True" w491 {
          tunnel: w490 -> [w496 _]
          frame False {
            n195 = Wait (ms)(milliseconds to wait=w496) -> ()  [unwired: 1 out]
          }
          frame True {
            # "If a message was received, immediately read again"
          }
        }
        n196 = shared-variable-read(w488, w489, 500 ("timeout ms")) -> (w486:errorcluster, w480:bool, →"CPU Usage (%)":dbl)  [unwired: 2 out]
        n197 = shared-variable-read(w487, w486) -> (w478:errorcluster, →"Free Memory (bytes)":dbl)  [unwired: 2 out]
        n198 = shared-variable-read(w479, w478) -> (w477:errorcluster, w476:T27)  [unwired: 2 out]
        n199 = Unbundle By Name(w476) -> ("TJM Temp"=→"Mandrel Temp":dbl, "BrgM Temp"=→"Brg Mandrel Temp":dbl, "Ambient Temp"=→"Ambient Temp":dbl, "Vessel Temp"=→"Vessel Temp":dbl)
        n200 = Index Array(array=w470) -> (element #1=→"NE":dbl, element #2=→"NW":dbl, element #3=→"SE":dbl, element #4=→"SW":dbl)  [unwired: 4 in]
        n201 = for {
          tunnel: w470 -> [w494] mode=indexing
          tunnel: [w493] -> w471 mode=indexing
          i -> [w495]
          n202 = Bundle(w495, "SW"=w494) -> (w493:cluster{i32, "SW":dbl})  [unwired: 1 in]
        }
        "Cylinder Force (lbf)" <- w471
        n203 = call "UI Error Handler - Monitoring.vi"("error in (no error)"=w477, "Lose Connection?"=w480, "Message Queue"=w481) -> ()  [unwired: 8 in, 1 out]
      }
    }
    n204 = global read "Global - All UI Loop Stop.vi" "All UI Loop Stop"() -> (w463:bool)
  }
  n205 = Unregister For Events(event registration refnum=w7, error in=w8) -> (error out=w6:errorcluster)
  n206 = Merge Errors(w6, w9) -> (w5:errorcluster)
  n207 = call "Destroy User Event - Stop.vi"("error in (no error)"=w5, "User Event - Stop"=w3) -> ("error out"=w4:errorcluster)  [unwired: 9 in]
  n208 = call <vilib>:"Simple Error Handler.vi"("error in (no error)"=w4) -> ()  [unwired: 4 in, 5 out]
